vi "SFPContinuous Processing and Trigger Detection.vi"(0 "Input Signals":waveform(dbl)[](array[waveform]), 7 "force trigger (F)":bool, 9 "status info in":variant, 11 "error in (no error)":errorcluster) -> (4 "signals":waveform(dbl)[](array[waveform]), 6 "signal available":bool, 8 "new trigger detected":bool, 10 "status info out":variant, 14 "trigger enabled":bool, 15 "error out":errorcluster)   [LabVIEW 2024, in "DSA_CFG_ACQ.lvlib"]
doc: "Continuous data processing is only done when the data exists AND no error. \n\nAll processes/measurements that need continuous data as input are done here. Waveform conditioning (filtering) and software triggering are two such processes. The order in which these are performed matters because both need continuous data as their inputs. Filtering outputs continuous stream of data while triggering outputs discontinuous blocks of data (one new block per detected trigger). Therefore, Filter is applied before Trigger Detection. \n\nAfter filtering and triggering are applied on the acquired data, data is stored into 'Block Data' queue. Note that 'Block Data' queue is a single-element queue. Use lossy enqueue element; the old time domain signal is overwritten by the new time domain signal. enqueue element would block the continuous processing loop until 'Block data' queue was emptied by BLOCK PROCESSING."
uses:
  DSA_CFG_ACQ.lvlib
  <vilib>/addons/_NISVFA/_Shared subVIs/Common/sv_Get NI Property Name String.vi
  <vilib>/addons/_NISVFA/_Shared subVIs/Common/sv_Get SV Property Name String.vi
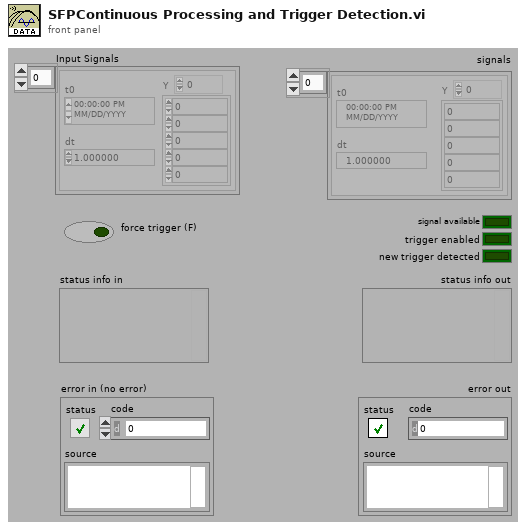
[diagram p1: front panel]
types:
  T1 = cluster{"level":dbl, "slope":u16, "hysteresis":dbl}
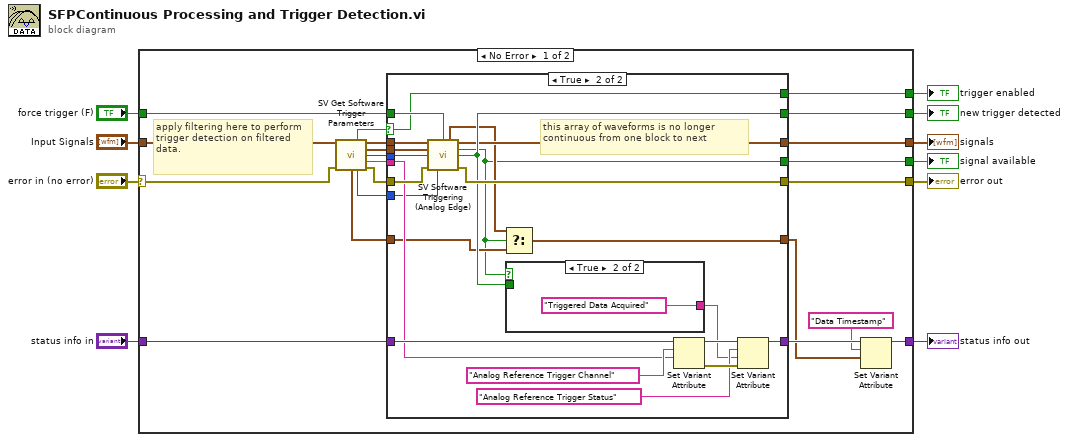
[diagram p0: block diagram]
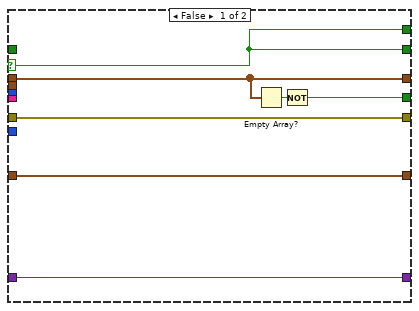
[diagram p2: hidden frame]
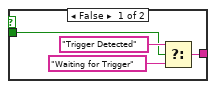
[diagram p3: hidden frame]
diagram:
  n1 = case shown="No Error" "error in (no error)" {
    selector: "error in (no error)" -> [w16 w68]
    tunnel: [w31 w68] -> w10
    tunnel: "Input Signals" -> [w17 w67]
    tunnel: [w30 w67] -> w7
    tunnel: [w29 _] -> w5
    tunnel: [w28 _] -> w4
    tunnel: "force trigger (F)" -> [w27 _]
    tunnel: [w25 w66] -> w3
    tunnel: "status info in" -> [w23 w66]
    tunnel: [w11 _] -> w1
    frame No Error {
      # "apply filtering here to perform trigger detection on filtered data."
      n2 = call <vilib>:"SV Get Software Trigger Parameters.vi"("scaled signals [EU] in"=w17, "error in"=w16) -> ("trigger channel found"=w18:bool, "scaled signals [EU] out"=w22:waveform(dbl)[], "level trigger configuration"=w14:T1, "trigger index"=w21:i32, "trigger channel name"=w19:string, "data timestamp"=w13:timestamp, "pretrigger samples"=w20:i32, "error out"=w15:errorcluster)  [unwired: 6 in]
      n3 = case "trigger signal found?" shown="True" w18 {
        selector: w18 -> [w32 w39]
        tunnel: w22 -> [w34 w48]
        tunnel: [w38 w59] -> w31
        tunnel: w15 -> [w38 w60]
        tunnel: w19 -> [_ w45]
        tunnel: w20 -> [_ w44]
        tunnel: [w36 w40] -> w29
        tunnel: [w32 w52] -> w28
        tunnel: [w34 w49] -> w30
        tunnel: w27 -> [_ w58]
        tunnel: w23 -> [w35 w51]
        tunnel: w21 -> [_ w46]
        tunnel: [w35 w50] -> w26
        tunnel: [w33 w47] -> w24
        tunnel: w13 -> [w33 w43]
        tunnel: w14 -> [_ w42]
        tunnel: [w32 w39] -> w11
        frame False {
          n4 = Empty Array?(array=w34) -> (empty?=w37:bool)
          n5 = Not(x=w37) -> (.not. x?=w36:bool)
        }
        frame True {
          # "this array of waveforms is no longer continuous from one block to next"
          n6 = call <vilib>:"SV Software Triggering (Analog Edge).vi"("input signals"=w48, "force trigger (F)"=w58, "level trigger configuration"=w42, "trigger channel index (0)"=w46, "error in (no error)"=w60, "pretrigger samples (0)"=w44) -> ("data timestamp"=w41:timestamp, "triggered signals"=w49:waveform(dbl)[], "output ready"=w40:bool, "new trigger detected"=w52:bool, "error out"=w59:errorcluster)  [unwired: 5 in]
          n7 = Select(t=w41, s=w40, f=w43) -> (s? t:f=w47:timestamp)
          n8 = case shown="True" w40 {
            tunnel: [w62 "Triggered Data Acquired" ("name")] -> w53
            tunnel: w52 -> [w61 _]
            frame False {
              n9 = Select(t="Trigger Detected" ("name"), s=w61, f="Waiting for Trigger" ("name")) -> (s? t:f=w62:string)
            }
            frame True {
            }
          }
          n10 = Set Variant Attribute(Variant=w51, name="Analog Reference Trigger Channel", value=w45) -> (Variant out=w56:variant, error out=w57:errorcluster)  [unwired: 1 in, 1 out]
          n11 = Set Variant Attribute(Variant=w56, name="Analog Reference Trigger Status", value=w53, error in=w57) -> (Variant out=w50:variant)  [unwired: 2 out]
        }
      }
      n12 = Set Variant Attribute(Variant=w26, name="Data Timestamp", value=w24) -> (Variant out=w25:variant)  [unwired: 1 in, 2 out]
    }
    frame Error {
    }
  }
  "error out" <- w10
  "signals" <- w7
  "signal available" <- w5
  "new trigger detected" <- w4
  "status info out" <- w3
  "trigger enabled" <- w1
